vi "fromXMLNative.vi"(8 "error in (no error)":errorcluster, 10 "xmlScript":refnum<k20>, 11 "DataPointScript in":refnum<class "DataPointScript.lvclass">) -> (0 "error out":errorcluster, 3 "DataPointScript out":refnum<class "DataPointScript.lvclass">)   [LabVIEW 2009, in "Tools.lvlib" / "Scripting.lvlib" / "DataPointScript.lvclass"]
uses:
  DataPointScript.lvclass
  ScriptingEvent/ScriptEventList/ScriptEventList.lvclass
  <vilib>/xml/Close Reference(Node).vi
  DataPointScript.lvclass/DataPointScript.ctl
  <vilib>/xml/NI_XML.lvlib
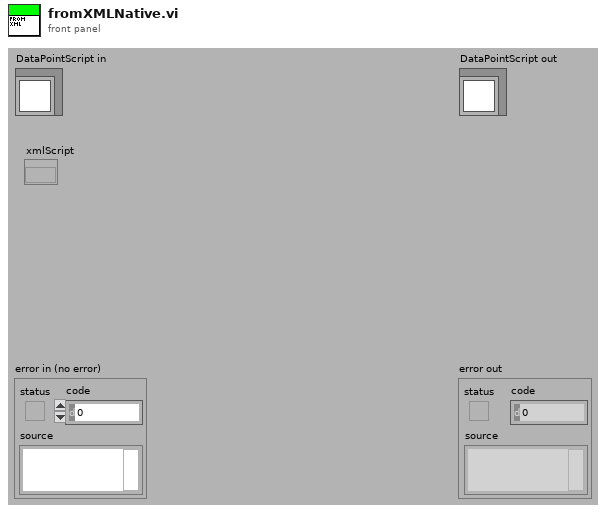
[diagram p1: front panel]
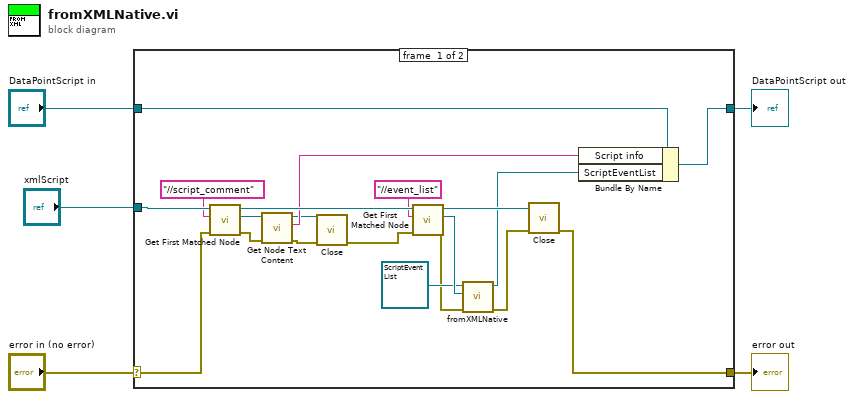
[diagram p0: block diagram]
diagram:
  n1 = case shown="No Error" "error in (no error)" {
    selector: "error in (no error)" -> [w11 w27]
    tunnel: [w15 w27] -> w4
    tunnel: [w12 w26] -> w2
    tunnel: "DataPointScript in" -> [w13 w26]
    tunnel: "xmlScript" -> [w25 _]
    frame #0 {
      n2 = call <vilib>:"Get First Matched Node.vi"("error in (no error)"=w11, "XPath expression"="//script_comment", "node in"=w25) -> ("error out"=w9:errorcluster, "node result"=w10:refnum<k20>, "node out"=w23:refnum<k20>)  [unwired: 6 in]
      n3 = call <vilib>:"Get Node Text Content.vi"("error in (no error)"=w9, "node in"=w10) -> ("error out"=w6:errorcluster, "node text"=w8:string, "node out"=w7:refnum<k20>)  [unwired: 7 in]
      n4 = call-poly <vilib>:"Close.vi"("error in (no error)"=w6, "node"=w7) -> ("error out"=w21:errorcluster)  [unwired: 7 in]
      n5 = call <vilib>:"Get First Matched Node.vi"("error in (no error)"=w21, "XPath expression"="//event_list", "node in"=w23) -> ("error out"=w17:errorcluster, "node result"=w20:refnum<k20>, "node out"=w16:refnum<k20>)  [unwired: 6 in]
      n6 = call "fromXMLNative.vi"("error in (no error)"=w17, "scriptEventListXML"=w20, "ScriptEventList in"=refnum<class "ScriptEventList.lvclass"> refnum) -> ("error out"=w19:errorcluster, "ScriptEventList out"=w14:refnum<class "ScriptEventList.lvclass">)  [unwired: 7 in]
      n7 = call-poly <vilib>:"Close.vi"("error in (no error)"=w19, "node"=w16) -> ("error out"=w15:errorcluster)  [unwired: 7 in]
      n8 = Bundle By Name(cluster=w13, "Script info"=w8, "ScriptEventList"=w14) -> (w12:refnum<class "DataPointScript.lvclass">)
    }
    frame #1 {
    }
  }
  "error out" <- w4
  "DataPointScript out" <- w2
